vi "Temperature Limit.vi"() -> ()   [LabVIEW 2015]
doc: "This VI simulates the acquisition of temperature, graphs the temperature, and notifies the user if the temperature is over the limit."
panel:
  in  "Start":bool
  in  "Delta t (ms)":i32(slide)=400 scale=50.0..500.0
  in  "Stop":bool
  in  "High Limit":dbl=28.0 format="%.2f"
  out "Temperature":cluster{"Temperature":dbl, "High Limit":dbl}(graph)={"Temperature"=85.88749999999999, "High Limit"=80.0}
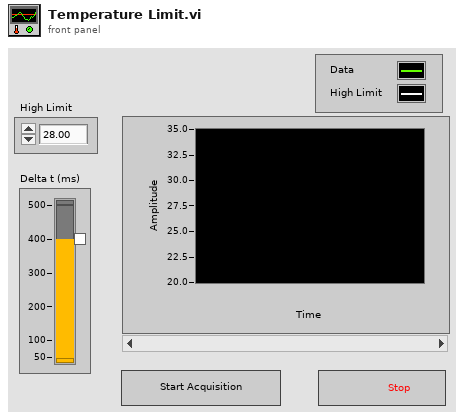
[diagram p1: front panel]
types:
  T1 = enum16{"Always On", "Always Off", "Off While Running"}
  T2 = cluster{"Temperature Value":dbl, "High Limit":dbl}
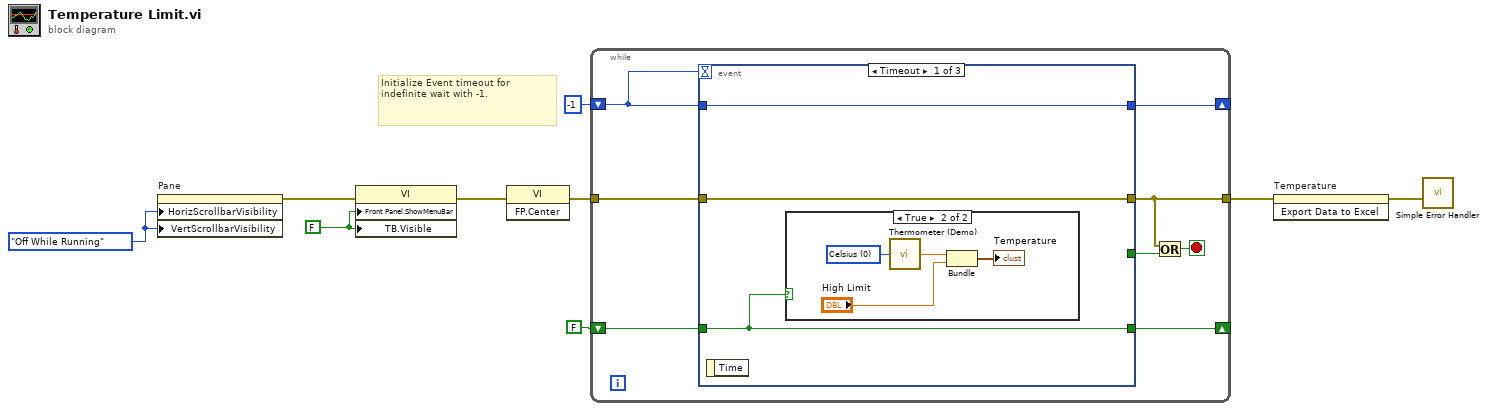
[diagram p0: block diagram]
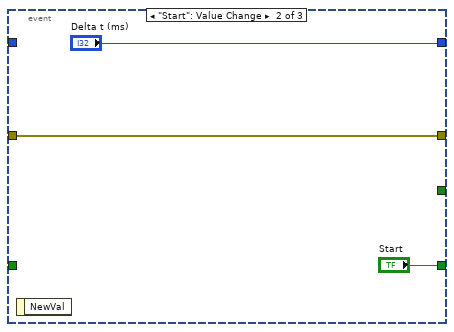
[diagram p3: hidden frame]
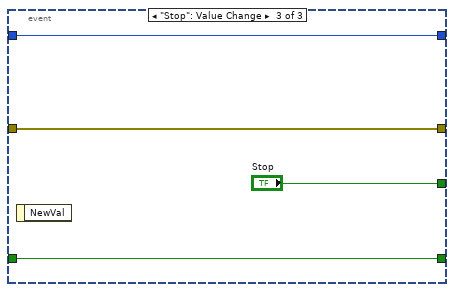
[diagram p4: hidden frame]
diagram:
  w6 = FALSE ("Tool Bar:Visible")
  w7 = T1."Off While Running" ("Vertical Scrollbar Visibility")
  # "Initialize Event timeout for indefinite wait with -1."
  n1 = property on="Pane" class="Pane"("HorizScrollbarVisibility"=w7, "VertScrollbarVisibility"=w7) -> (error out=w5:errorcluster)  [unwired: 2 in, 1 out]
  n2 = property class="VI"(error in=w5, "Front Panel.ShowMenuBar"=w6, "TB.Visible"=w6) -> (error out=w3:errorcluster)  [unwired: 1 in, 1 out]
  n3 = invoke class="VI" method="FP.Center"(error in=w3) -> (error out=w4:errorcluster)  [unwired: 2 in, 2 out]
  n4 = while {
    tunnel: w4 -> [w17]
    tunnel: [w15] -> w2
    shift-right: [w13] -> _
    shift-left: FALSE ("Start") -> [w12]
    shift-right: [w11] -> _
    shift-left: -1 ("Delta t (ms)") -> [w10]
    stop <- w16 stop-if-true
    n5 = event shown="[0] Timeout" {
      selector: _ -> [_ _ _]
      dyn-events: _ -> [_ _ _]
      timeout: w10 -> [_ _ _]
      tunnel: [_ _ "Stop"] -> w14
      tunnel: w17 -> [w20 w25 w30]
      tunnel: [w20 w25 w30] -> w15
      tunnel: [w18 "Start" w29] -> w13
      tunnel: w12 -> [w18 _ w29]
      tunnel: [w19 "Delta t (ms)" w28] -> w11
      tunnel: w10 -> [w19 _ w28]
      event Timeout {
        n6 = event-data() -> ()  [unwired: 1 in, 1 out]
        n7 = case shown="True" w18 {
          frame False {
          }
          frame True {
            w21 = u16 0 items=["Celsius", "Fahrenheit"] ("Units (0: Celsius)")
            n8 = call "Thermometer (Demo).vi"("Units (0: Celsius)"=w21) -> ("Temperature Value"=w22:dbl)
            n9 = Bundle("Temperature Value"=w22, "High Limit"="High Limit") -> (→"Temperature":T2)  [unwired: 1 in]
          }
        }
      }
      event "Start": Value Change {
        n10 = event-data() -> ()  [unwired: 1 in, 1 out]
      }
      event "Stop": Value Change {
        n11 = event-data() -> ()  [unwired: 1 in, 1 out]
      }
    }
    n12 = Or(x=w15, y=w14) -> (x .or. y?=w16:bool)
  }
  n13 = invoke on="Temperature" class="WFChart (strict)" method="Export Data to Excel"(error in=w2) -> (error out=w1:errorcluster)  [unwired: 2 in, 2 out]
  n14 = call <vilib>:"Simple Error Handler.vi"("error in (no error)"=w1) -> ()  [unwired: 4 in, 5 out]
